vi "FunctDataMgr.Update Test Mode.vi"(8 "error in (no error)":errorcluster, 10 "Mode":string, 11 "FunctDataMgr in":refnum<class "FunctDataMgr.lvclass">) -> (0 "error out":errorcluster, 3 "FunctDataMgr out":refnum<class "FunctDataMgr.lvclass">)   [LabVIEW 2018, in "FunctDataMgr.lvclass"]
uses:
  FunctDataMgr.lvclass
  FunctDataMgr.lvclass/FunctDataMgr.ctl
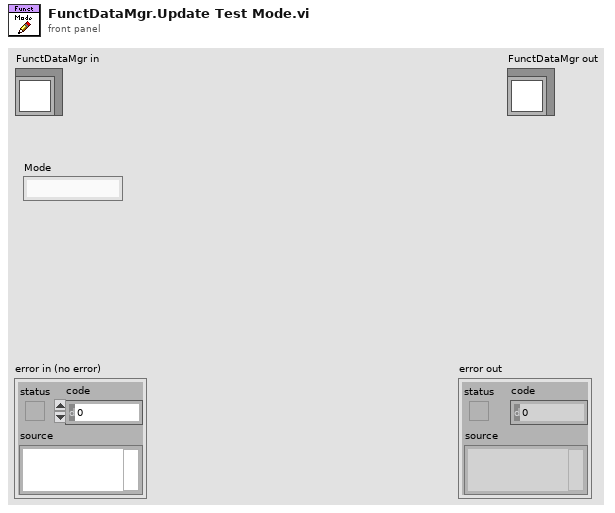
[diagram p1: front panel]
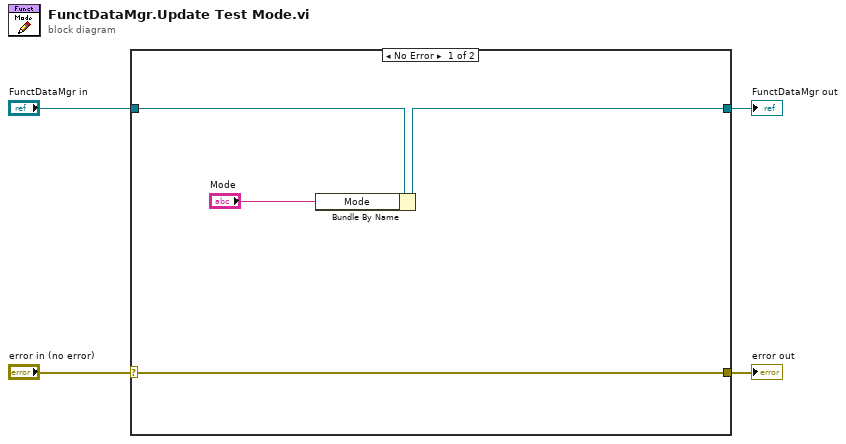
[diagram p0: block diagram]
diagram:
  n1 = case shown="No Error" "error in (no error)" {
    selector: "error in (no error)" -> [w8 w10]
    tunnel: [w8 w10] -> w3
    tunnel: [w6 w9] -> w1
    tunnel: "FunctDataMgr in" -> [w7 w9]
    frame No Error {
      n2 = Bundle By Name(cluster=w7, "Mode"="Mode") -> (w6:refnum<class "FunctDataMgr.lvclass">)
    }
    frame Error {
    }
  }
  "error out" <- w3
  "FunctDataMgr out" <- w1
